vi "CreateSourceDirectory.vi"(8 "error in":errorcluster, 11 "RasPi Compiler in":refnum<class "RasPi Compiler.lvclass">) -> (0 "error out":errorcluster, 3 "RasPi Compiler out":refnum<class "RasPi Compiler.lvclass">)   [LabVIEW 2014, in "Raspberry Pi Compatible Compiler for LabVIEW.lvlib" / "RasPi Compiler.lvclass"]
uses:
  RasPi Compiler.lvclass
  RasPi Compiler.lvclass/RasPi Compiler.ctl
  VI Interpreter/Classes/VI Interpreter/VI Interpreter.lvclass
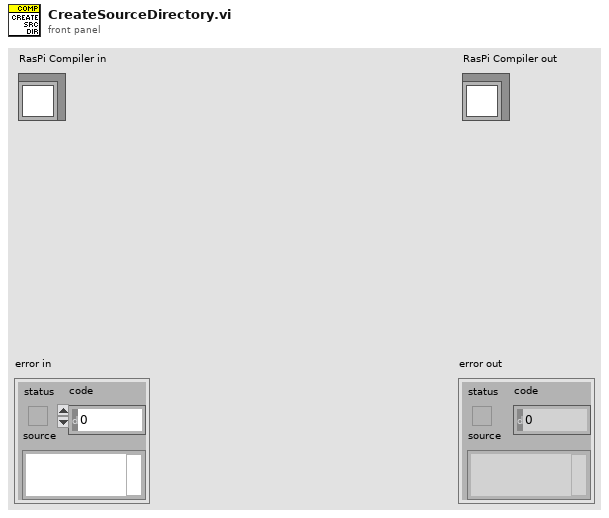
[diagram p1: front panel]
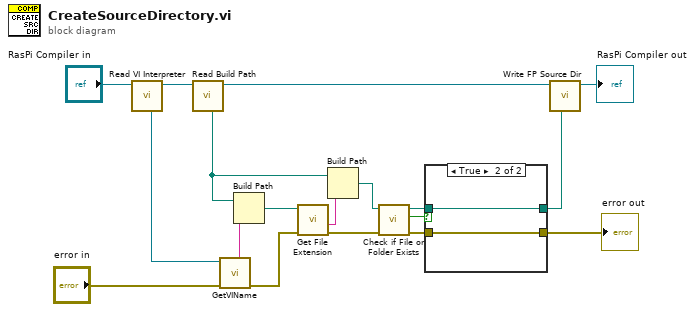
[diagram p0: block diagram]
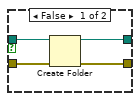
[diagram p2: hidden frame]
diagram:
  n1 = call "Read VI Interpreter.vi"("RasPi Compiler in"="RasPi Compiler in") -> ("RasPi Compiler out"=w2:refnum<class "RasPi Compiler.lvclass">, "VI Interpreter"=w10:refnum<class "VI Interpreter.lvclass">)  [unwired: 7 in]
  n2 = call "Read Build Path.vi"("RasPi Compiler in"=w2) -> ("RasPi Compiler out"=w1:refnum<class "RasPi Compiler.lvclass">, "Build Path"=w3:path)  [unwired: 7 in]
  n3 = call "GetVIName.vi"("error in"="error in", "VI Interpreter in"=w10) -> ("error out"=w8:errorcluster, "VI Name"=w12:string)  [unwired: 5 in, 1 out]
  n4 = Build Path(base path=w3, name or relative path=w12) -> (appended path=w13:path)
  n5 = call <vilib>:"Get File Extension.vi"("error in (no error)"=w8, "file"=w13) -> ("error out"=w7:errorcluster, "filename without extension"=w14:string)  [unwired: 6 in, 2 out]
  n6 = Build Path(base path=w3, name or relative path=w14) -> (appended path=w11:path)
  n7 = call <vilib>:"Check if File or Folder Exists.vi"("error in (no error)"=w7, "path"=w11) -> ("error out"=w16:errorcluster, "file or folder exists?"=w17:bool, "dup path"=w15:path)  [unwired: 7 in]
  n8 = case shown="True" w17 {
    tunnel: w15 -> [w22 w23]
    tunnel: w16 -> [w21 w24]
    tunnel: [w20 w24] -> w4
    tunnel: [w19 w23] -> w6
    frame False {
      n9 = Create Folder(path (use dialog)=w22, error in=w21) -> (created path=w19:path, error out=w20:errorcluster)  [unwired: 1 in, 1 out]
    }
    frame True {
    }
  }
  "error out" <- w4
  n10 = call "Write FP Source Dir.vi"("FP Source Dir"=w6, "RasPi Compiler in"=w1) -> ("RasPi Compiler out"=→"RasPi Compiler out":refnum<class "RasPi Compiler.lvclass">)  [unwired: 7 in]
